vi "WindowParams.vi"(8 "error in (no error)":errorcluster, 11 "RingdownPlugin":refnum<class "RingdownPlugin.lvclass">) -> (0 "error out":errorcluster, 3 "RingdownPlugin.lvclass":refnum<class "RingdownPlugin.lvclass">)   [LabVIEW 2014, in "AppPlugins.lvlib" / "RingdownPlugin.lvclass"]
uses:
  RingdownPlugin.lvclass
  AppPluginBaseClass/AppPluginsBase.lvclass/AppPluginsBase.ctl
  RingdownPlugin.lvclass/RingdownPlugin.ctl
  AppPluginBaseClass/Accessors/Read clEvtReportArray.vi
  Accessors/Read RingdownConfig.vi
  Accessors/Write RingdownConfig.vi
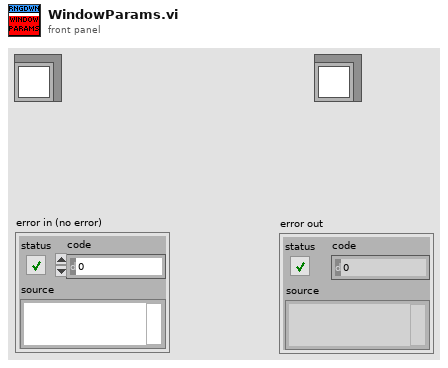
[diagram p1: front panel]
types:
  T1 = typedef "EventPlugins.lvlib/EventPluginBaseClass.lvclass/clEvtReportArray.ctl" = T2[]
  T2 = typedef "EventPlugins.lvlib/EventPluginBaseClass.lvclass/clEvtReport.ctl" = cluster{"Timestamp":dbl, "Synx":cdb[], "Freq":dbl, "ROCOF":dbl, "ID":i16}
  T3 = typedef "AppPlugins.lvlib/RingdownPlugin.lvclass/RingdownConfig.ctl" = cluster{"Config":cluster{"Addmod":i32, "Scalmod":i32, "Lpocon":i32, "Pircon":i32, "Dmodes":i32, "Lpmcon":u16, "Lpacon":u16, "Fbcon":u16, "Ordcon":i32, "Trimre":dbl, "Ftrimh":dbl, "Ftriml":dbl}, "Window":cluster{"StOffset":i32, "EndOffset":i32, "Length":i32}, "V index":i32, "I index":i32, "PosSeq":bool}
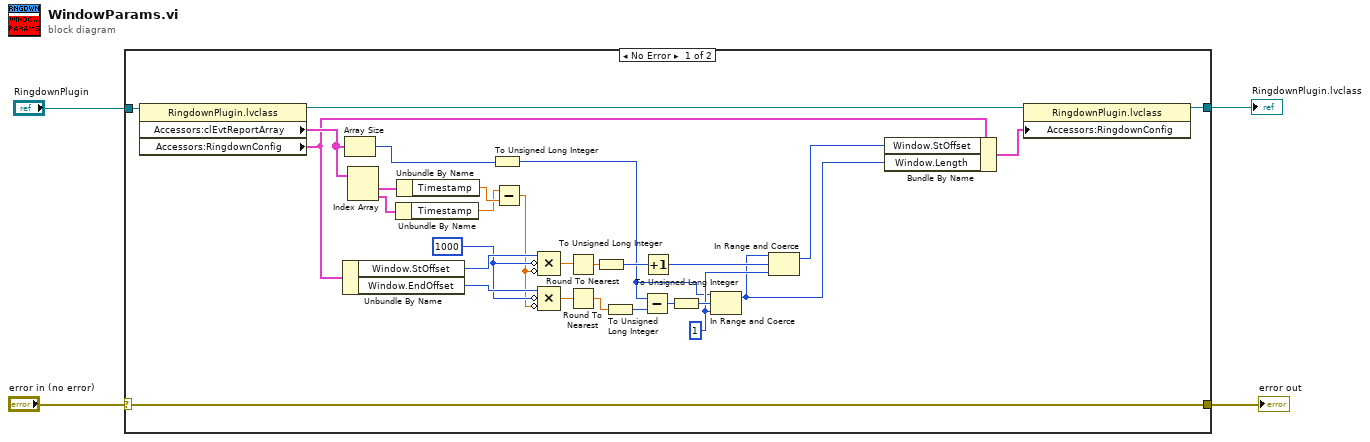
[diagram p0: block diagram]
diagram:
  n1 = case shown="No Error" "error in (no error)" {
    selector: "error in (no error)" -> [w32 w35]
    tunnel: [w32 w35] -> w3
    tunnel: "RingdownPlugin" -> [w33 w34]
    tunnel: [w8 w34] -> w1
    frame No Error {
      w14 = u32 1 ("lower limit")
      w24 = 1000
      n2 = property class="RingdownPlugin.lvclass"(reference=w33) -> (reference out=w11:refnum<class "RingdownPlugin.lvclass">, "Accessors:clEvtReportArray"=w27:T1, "Accessors:RingdownConfig"=w10:T3)  [unwired: 1 in, 1 out]
      n3 = Unbundle By Name(w10) -> ("Window.StOffset"=w26:i32, "Window.EndOffset"=w25:i32)
      n4 = Array Size(array=w27) -> (size(s)=w19:i32)
      n5 = Index Array(array=w27) -> (element #1=w31:T2, element #2=w30:T2)  [unwired: 2 in]
      n6 = Unbundle By Name(w30) -> ("Timestamp"=w28:dbl)
      n7 = Unbundle By Name(w31) -> ("Timestamp"=w29:dbl)
      n8 = To Unsigned Long Integer(number=w19) -> (unsigned 32bit integer=w7:u32)
      n9 = Subtract(x=w28, y=w29) -> (x-y=w18:dbl)
      n10 = Compound Arithmetic op=MULTIPLY(w26, invert w24, invert w18) -> (w23:dbl)
      n11 = Compound Arithmetic op=MULTIPLY(w25, invert w24, invert w18) -> (w22:dbl)
      n12 = Round To Nearest(number=w23) -> (nearest integer value=w21:dbl)
      n13 = Round To Nearest(number=w22) -> (nearest integer value=w6:dbl)
      n14 = To Unsigned Long Integer(number=w21) -> (unsigned 32bit integer=w20:u32)
      n15 = To Unsigned Long Integer(number=w6) -> (unsigned 32bit integer=w5:u32)
      n16 = Subtract(x=w7, y=w5) -> (x-y=w17:u32)
      n17 = Increment(x=w20) -> (x+1=w15:u32)
      n18 = To Unsigned Long Integer(number=w17) -> (unsigned 32bit integer=w16:u32)
      n19 = In Range and Coerce(upper limit=w7, x=w16, lower limit=w14) -> (coerced(x)=w13:u32)  [unwired: 1 out]
      n20 = In Range and Coerce(upper limit=w13, x=w15, lower limit=w14) -> (coerced(x)=w12:u32)  [unwired: 1 out]
      n21 = Bundle By Name(cluster=w10, "Window.StOffset"=w12, "Window.Length"=w13) -> (w9:T3)
      n22 = property class="RingdownPlugin.lvclass"(reference=w11, "Accessors:RingdownConfig"=w9) -> (reference out=w8:refnum<class "RingdownPlugin.lvclass">)  [unwired: 1 in, 1 out]
    }
    frame Error {
    }
  }
  "RingdownPlugin.lvclass" <- w1
  "error out" <- w3
